vi "HFRR ADV v015 new software.vi"() -> ()   [LabVIEW 2025] (continued)
            n3529 = property class="DigNum (strict)"("Numeric Text.Text Colors:BG Color"="NC BG") -> ()  [unwired: 2 in, 2 out]
            n3530 = property class="DigNum (strict)"("Numeric Text.Text Colors:BG Color"="NC BG") -> ()  [unwired: 2 in, 2 out]
            n3531 = property class="DigNum (strict)"("Numeric Text.Text Colors:BG Color"="NC BG") -> ()  [unwired: 2 in, 2 out]
            n3532 = property class="DigNum (strict)"("Numeric Text.Text Colors:BG Color"="NC BG") -> ()  [unwired: 2 in, 2 out]
            n3533 = property class="DigNum (strict)"("Numeric Text.Text Colors:BG Color"="NC BG") -> ()  [unwired: 2 in, 2 out]
            n3534 = property class="DigNum (strict)"("Numeric Text.Text Colors:BG Color"="NC BG") -> ()  [unwired: 2 in, 2 out]
            n3535 = property class="DigNum (strict)"("Numeric Text.Text Colors:BG Color"="NC BG") -> ()  [unwired: 2 in, 2 out]
            n3536 = property class="DigNum (strict)"("Numeric Text.Text Colors:BG Color"="NC BG") -> ()  [unwired: 2 in, 2 out]
            n3537 = property class="DigNum (strict)"("Numeric Text.Text Colors:BG Color"="NC BG") -> ()  [unwired: 2 in, 2 out]
            n3538 = property class="DigNum (strict)"("Numeric Text.Text Colors:BG Color"="NC BG") -> ()  [unwired: 2 in, 2 out]
            n3539 = property class="DigNum (strict)"("Numeric Text.Text Colors:BG Color"="NC BG") -> ()  [unwired: 2 in, 2 out]
            n3540 = property on="FILE" class="Str"("Text.Text Colors:BG Color"="SC BG 3") -> ()  [unwired: 2 in, 2 out]
            n3541 = property on="Fuel Discription :" class="Str"("Text.Text Colors:BG Color"="SC BG 3") -> ()  [unwired: 2 in, 2 out]
            n3542 = property on="tested by" class="Str"("Text.Text Colors:BG Color"="SC BG 3") -> ()  [unwired: 2 in, 2 out]
            n3543 = property on="Remarks :" class="Str"("Text.Text Colors:BG Color"="SC BG 3") -> ()  [unwired: 2 in, 2 out]
            n3544 = property class="DigNum (strict)"("Numeric Text.Text Colors:Text Color"="NC Text") -> ()  [unwired: 2 in, 2 out]
            n3545 = property class="DigNum (strict)"("Numeric Text.Text Colors:Text Color"="NC Text") -> ()  [unwired: 2 in, 2 out]
            n3546 = property class="DigNum (strict)"("Numeric Text.Text Colors:Text Color"="NC Text") -> ()  [unwired: 2 in, 2 out]
            n3547 = property class="DigNum (strict)"("Numeric Text.Text Colors:Text Color"="NC Text") -> ()  [unwired: 2 in, 2 out]
            n3548 = property class="DigNum (strict)"("Numeric Text.Text Colors:Text Color"="NC Text") -> ()  [unwired: 2 in, 2 out]
            n3549 = property class="DigNum (strict)"("Numeric Text.Text Colors:Text Color"="NC Text") -> ()  [unwired: 2 in, 2 out]
            n3550 = property class="DigNum (strict)"("Numeric Text.Text Colors:Text Color"="NC Text") -> ()  [unwired: 2 in, 2 out]
            n3551 = property class="DigNum (strict)"("Numeric Text.Text Colors:Text Color"="NC Text") -> ()  [unwired: 2 in, 2 out]
            n3552 = property class="DigNum (strict)"("Numeric Text.Text Colors:Text Color"="NC Text") -> ()  [unwired: 2 in, 2 out]
            n3553 = property class="DigNum (strict)"("Numeric Text.Text Colors:Text Color"="NC Text") -> ()  [unwired: 2 in, 2 out]
            n3554 = property class="DigNum (strict)"("Numeric Text.Text Colors:Text Color"="NC Text") -> ()  [unwired: 2 in, 2 out]
            n3555 = property class="DigNum (strict)"("Numeric Text.Text Colors:Text Color"="NC Text") -> ()  [unwired: 2 in, 2 out]
            n3556 = property class="DigNum (strict)"("Numeric Text.Text Colors:Text Color"="NI Text  2") -> ()  [unwired: 2 in, 2 out]
            n3557 = property class="DigNum (strict)"("Numeric Text.Text Colors:Text Color"="NI Text  2") -> ()  [unwired: 2 in, 2 out]
            n3558 = property class="DigNum (strict)"("Numeric Text.Text Colors:Text Color"="NI Text  2") -> ()  [unwired: 2 in, 2 out]
            n3559 = property class="DigNum (strict)"("Numeric Text.Text Colors:Text Color"="NI Text  2") -> ()  [unwired: 2 in, 2 out]
            n3560 = property class="DigNum (strict)"("Numeric Text.Text Colors:Text Color"="NI Text  2") -> ()  [unwired: 2 in, 2 out]
            n3561 = property class="DigNum (strict)"("Numeric Text.Text Colors:Text Color"="NI Text  2") -> ()  [unwired: 2 in, 2 out]
            n3562 = property class="DigNum (strict)"("Numeric Text.Text Colors:Text Color"="NI Text  2") -> ()  [unwired: 2 in, 2 out]
            n3563 = property class="DigNum (strict)"("Numeric Text.Text Colors:Text Color"="NI Text  2") -> ()  [unwired: 2 in, 2 out]
            n3564 = property class="DigNum (strict)"("Numeric Text.Text Colors:Text Color"="NI Text  2") -> ()  [unwired: 2 in, 2 out]
            n3565 = property class="DigNum (strict)"("Numeric Text.Text Colors:Text Color"="NI Text  2") -> ()  [unwired: 2 in, 2 out]
            n3566 = property class="DigNum (strict)"("Numeric Text.Text Colors:Text Color"="NI Text  2") -> ()  [unwired: 2 in, 2 out]
            n3567 = property class="DigNum (strict)"("Numeric Text.Text Colors:Text Color"="NI Text  2") -> ()  [unwired: 2 in, 2 out]
            n3568 = property class="DigNum (strict)"("Numeric Text.Text Colors:Text Color"="NI Text  2") -> ()  [unwired: 2 in, 2 out]
            n3569 = property class="DigNum (strict)"("Numeric Text.Text Colors:Text Color"="NI Text  2") -> ()  [unwired: 2 in, 2 out]
            n3570 = property class="DigNum (strict)"("Numeric Text.Text Colors:Text Color"="NI Text  2") -> ()  [unwired: 2 in, 2 out]
            n3571 = property on="Coefficient Of Friction" class="XYGraph (strict)"("Plot Area:Colors:FG Color"="GFG  2", "Plot Area:Colors:BG Color"="GBG   2") -> ()  [unwired: 2 in, 2 out]
            n3572 = property on="Humidity ( %RH )" class="XYGraph (strict)"("Plot Area:Colors:FG Color"="GFG  2", "Plot Area:Colors:BG Color"="GBG   2") -> ()  [unwired: 2 in, 2 out]
            n3573 = property on="Air Temperature  ( °C )" class="XYGraph (strict)"("Plot Area:Colors:FG Color"="GFG  2", "Plot Area:Colors:BG Color"="GBG   2") -> ()  [unwired: 2 in, 2 out]
            n3574 = property on="Sample Temperature ( °C )" class="XYGraph (strict)"("Plot Area:Colors:FG Color"="GFG  2", "Plot Area:Colors:BG Color"="GBG   2") -> ()  [unwired: 2 in, 2 out]
            n3575 = property class="DigNum (strict)"("Numeric Text.Text Colors:BG Color"="NI BG 2") -> ()  [unwired: 2 in, 2 out]
            n3576 = property class="DigNum (strict)"("Numeric Text.Text Colors:BG Color"="NI BG 2") -> ()  [unwired: 2 in, 2 out]
            n3577 = property class="DigNum (strict)"("Numeric Text.Text Colors:BG Color"="NI BG 2") -> ()  [unwired: 2 in, 2 out]
            n3578 = property class="DigNum (strict)"("Numeric Text.Text Colors:BG Color"="NI BG 2") -> ()  [unwired: 2 in, 2 out]
            n3579 = property class="DigNum (strict)"("Numeric Text.Text Colors:BG Color"="NI BG 2") -> ()  [unwired: 2 in, 2 out]
            n3580 = property class="DigNum (strict)"("Numeric Text.Text Colors:BG Color"="NI BG 2") -> ()  [unwired: 2 in, 2 out]
            n3581 = property class="DigNum (strict)"("Numeric Text.Text Colors:BG Color"="NI BG 2") -> ()  [unwired: 2 in, 2 out]
            n3582 = property class="DigNum (strict)"("Numeric Text.Text Colors:BG Color"="NI BG 2") -> ()  [unwired: 2 in, 2 out]
            n3583 = property class="DigNum (strict)"("Numeric Text.Text Colors:BG Color"="NI BG 2") -> ()  [unwired: 2 in, 2 out]
            n3584 = property class="DigNum (strict)"("Numeric Text.Text Colors:BG Color"="NI BG 2") -> ()  [unwired: 2 in, 2 out]
            n3585 = property class="DigNum (strict)"("Numeric Text.Text Colors:BG Color"="NI BG 2") -> ()  [unwired: 2 in, 2 out]
            n3586 = property class="DigNum (strict)"("Numeric Text.Text Colors:BG Color"="NI BG 2") -> ()  [unwired: 2 in, 2 out]
            n3587 = property class="DigNum (strict)"("Numeric Text.Text Colors:BG Color"="NI BG 2") -> ()  [unwired: 2 in, 2 out]
            n3588 = property class="DigNum (strict)"("Numeric Text.Text Colors:BG Color"="NI BG 2") -> ()  [unwired: 2 in, 2 out]
            n3589 = property class="DigNum (strict)"("Numeric Text.Text Colors:BG Color"="NI BG 2") -> ()  [unwired: 2 in, 2 out]
            n3590 = property class="Bool"("Colors [4]"="Boolean BC T & BG") -> ()  [unwired: 2 in, 2 out]
            n3591 = property on="Save & Continue" class="Bool (strict)"("Colors [4]"="Boolean BC T & BG") -> ()  [unwired: 2 in, 2 out]
            n3592 = property on="Heater Button" class="Bool (strict)"("Colors [4]"="Boolean BC T & BG") -> ()  [unwired: 2 in, 2 out]
            n3593 = property class="Bool"("Colors [4]"="Boolean BC T & BG") -> ()  [unwired: 2 in, 2 out]
            n3594 = property on="Humidity" class="Bool (strict)"("Colors [4]"="Boolean BC T & BG") -> ()  [unwired: 2 in, 2 out]
            n3595 = property class="Bool (strict)"("Colors [4]"="Boolean BC T & BG") -> ()  [unwired: 2 in, 2 out]
            n3596 = property on="RUN" class="Bool (strict)"("Colors [4]"="Boolean BC T & BG") -> ()  [unwired: 2 in, 2 out]
            n3597 = property on="trip1 8" class="Bool (strict)"("Colors [4]"="Boolean BC T & BG") -> ()  [unwired: 2 in, 2 out]
            n3598 = property class="Bool"("Colors [4]"="Boolean BC T & BG") -> ()  [unwired: 2 in, 2 out]
            n3599 = property class="Bool (strict)"("Colors [4]"="Boolean BC T & BG") -> ()  [unwired: 2 in, 2 out]
            n3600 = property on="OPEN 1" class="Bool (strict)"("Colors [4]"="Boolean BC T & BG 2") -> ()  [unwired: 2 in, 2 out]
            n3601 = property on="OPEN 2" class="Bool (strict)"("Colors [4]"="Boolean BC T & BG 2") -> ()  [unwired: 2 in, 2 out]
            n3602 = property on="OPEN 3" class="Bool (strict)"("Colors [4]"="Boolean BC T & BG 2") -> ()  [unwired: 2 in, 2 out]
            n3603 = property on="OPEN 4" class="Bool (strict)"("Colors [4]"="Boolean BC T & BG 2") -> ()  [unwired: 2 in, 2 out]
            n3604 = property on="OPEN" class="Bool (strict)"("Colors [4]"="Boolean BC T & BG 2") -> ()  [unwired: 2 in, 2 out]
            n3605 = property on="rstv2" class="Bool"("Colors [4]"="Boolean BC T & BG 2") -> ()  [unwired: 2 in, 2 out]
            n3606 = property on="RST CP" class="Bool"("Colors [4]"="Boolean BC T & BG 2") -> ()  [unwired: 2 in, 2 out]
            n3607 = property on="RSTV1 3" class="Bool"("Colors [4]"="Boolean BC T & BG 2") -> ()  [unwired: 2 in, 2 out]
            n3608 = property on="RSTV1 2" class="Bool"("Colors [4]"="Boolean BC T & BG 2") -> ()  [unwired: 2 in, 2 out]
          }
          frame #1 {
          }
        }
        n3609 = local read "Quit"() -> (w4479:bool)
      }
    }
    frame Enabled {
    }
  }
  n3610 = while {
    shift-right: [w4497] -> _
    shift-left: _ -> [w4498]
    shift-right: [w4495] -> _
    shift-left: T19 {"Read Heave and Surge"="", "Bytes at Heave Port"=0.0, "Heave and Surge COM Port:"="COM9", "Com Port 2"="COM7", "Residual Due"="", "Heave COM Status 2"=TRUE, "Heave COM Status"=TRUE, "Port 2"=TRUE, "Sway PPR"=6400.0, "Surge PPR"=6400.0, "Heave PPR"=6400.0, "Sway Pitch"=2.0, "Surge Pitch"=3.0, "Heave Pitch"=4.0, "Sway Pulses/mm"=320.0, "Surge Pulses/mm"=1600.0, "Heave Pulses/mm"=1600.0, "inner loop"=0.0, "Read Heave and Surge 2"="", "String 36"="", "Write S"=FALSE, "WriteCC1"=[""], "Heave COM Loop"=0, "LastCom"="", "EXIT"=FALSE, "Error Heave"={"status"=TRUE, "code"=-1073807343, "source"=""}} -> [w4494]
    shift-right: [w4492] -> _
    shift-left: enum16{"init", "MAIN", "Panel Close"}."init" -> [w4493]
    stop <- w4496 stop-if-true
    n3611 = case shown="\"MAIN\"" w4493 {
      tunnel: w4498 -> [w4512 w4527 w4588 w4590]
      tunnel: [w4506 w4536 w4588 w4590] -> w4497
      tunnel: [_ _ TRUE _] -> w4496
      tunnel: [w4502 w4533 w4586 w4589] -> w4495
      tunnel: w4494 -> [w4509 w4526 w4586 w4589]
      tunnel: [enum16{"init", "MAIN", "Panel Close"}."MAIN" w4520 _ _] -> w4492
      frame "init" {
        n3612 = Bundle By Name(cluster=w4509, "Heave and Surge COM Port:"="C3 :") -> (w4508:T19)
        n3613 = call "Instrument fgv.vi"("Enum"=T31."INIT", "error in (no error) 2"=w4512, "INPUT"=w4508) -> ("error"=w4510:errorcluster, "output"=w4505:T19)  [unwired: 6 in, 1 out]
        n3614 = case shown="Error" w4510 {
          selector: w4510 -> [w4514 _]
          tunnel: [w4514 w4518] -> w4506
          tunnel: w4505 -> [w4513 w4516]
          tunnel: [w4513 w4515] -> w4503
          frame No Error {
          }
          frame Error {
            n3615 = call "Instrument fgv.vi"("Enum"=T31."ERROR INIT", "INPUT"=w4516) -> ("error"=w4519:errorcluster, "output"=w4515:T19)  [unwired: 7 in, 1 out]
            n3616 = call <vilib>:"Clear Errors.vi"("error in (no error)"=w4519) -> ("error out"=w4518:errorcluster)  [unwired: 5 in, 1 out]
          }
        }
        n3617 = local read "LastCom"() -> (w4501:string)
        n3618 = Unbundle By Name(w4503) -> ("Heave COM Status 2"=→"COM Status" →"Instrument Status":bool, "Error Heave"=→"Error":errorcluster)  [unwired: 1 out]
        n3619 = Bundle By Name(cluster=w4503, "LastCom"=w4501) -> (w4502:T19)
      }
      frame "MAIN" {
        n3620 = Unbundle By Name(w4526) -> ("Com Port 2"=w4538:refnum<visa-resource-name>)
        n3621 = local write "Com Port 4"(w4538) -> ()
        n3622 = local read "C3 :"() -> (w4524:refnum<visa-resource-name>)
        n3623 = Bundle By Name(cluster=w4526, "Heave and Surge COM Port:"=w4524) -> (w4525:T19)
        n3624 = Equal?(x=w4538, y=w4524) -> (x = y?=w4537:bool)
        n3625 = case shown="True" w4537 {
          tunnel: [w4542 w4559] -> w4536
          tunnel: w4527 -> [w4543 w4565]
          tunnel: w4525 -> [w4541 w4563]
          tunnel: [w4540 w4558] -> w4533
          frame False {
            n3626 = call <vilib>:"Clear Errors.vi"("error in (no error)"=w4543) -> ("error out"=w4539:errorcluster)  [unwired: 5 in, 1 out]
            n3627 = call "Instrument fgv.vi"("Enum"=T31."ERROR INIT", "error in (no error) 2"=w4539, "INPUT"=w4541) -> ("error"=w4545:errorcluster, "output"=w4540:T19)  [unwired: 6 in, 1 out]
            n3628 = call <vilib>:"Clear Errors.vi"("error in (no error)"=w4545) -> ("error out"=w4542:errorcluster)  [unwired: 5 in, 1 out]
          }
          frame True {
            n3629 = call "Instrument fgv.vi"("Enum"=T31."READ", "error in (no error) 2"=w4565, "INPUT"=w4563) -> ("error"=w4564:errorcluster, "output"=w4555:T19)  [unwired: 6 in, 1 out]
            n3630 = Bundle By Name(cluster=w4555, "String 36"="String 11") -> (w4554:T19)
            n3631 = case shown="True" "Write S" {
              selector: "Write S" -> [_ w4585]
              tunnel: w4564 -> [w4578 w4584]
              tunnel: [w4578 w4583] -> w4551
              tunnel: w4554 -> [w4577 w4580]
              tunnel: [w4577 w4579] -> w4550
              frame False {
              }
              frame True {
                n3632 = Not(x=w4585) -> (.not. x?=w4581:bool)
                n3633 = local write "Write S"(w4581) -> ()
                n3634 = call "Instrument fgv.vi"("Enum"=T31."MANUAL WRITE", "error in (no error) 2"=w4584, "INPUT"=w4580) -> ("error"=w4583:errorcluster, "output"=w4579:T19)  [unwired: 6 in, 1 out]
              }
            }
            n3635 = Array Size(array="WriteHumidity") -> (size(s)=w4548:i32)
            n3636 = Greater Than 0?(x=w4548) -> (x > 0?=w4546:bool)
            n3637 = call "Instrument fgv.vi"("Enum"=T31."WRITE", "error in (no error) 2"=w4551, "WriteCC1"="WriteHumidity", "INPUT"=w4550) -> ("error"=w4561:errorcluster, "WriteCC1 2"=w4549:string[], "output"=w4560:T19)  [unwired: 5 in]
            n3638 = case shown="True" w4546 {
              tunnel: w4549 -> [_ w4567]
              frame False {
              }
              frame True {
                n3639 = local write "WriteHumidity"(w4567) -> ()
              }
            }
            n3640 = case shown="Error" w4561 {
              selector: w4561 -> [w4568 w4571]
              tunnel: w4560 -> [w4569 w4576]
              tunnel: [w4569 w4575] -> w4558
              tunnel: [w4568 w4573] -> w4559
              frame No Error {
              }
              frame Error {
                n3641 = call <vilib>:"Clear Errors.vi"("error in (no error)"=w4571) -> ("error out"=w4570:errorcluster)  [unwired: 5 in, 1 out]
                n3642 = call "Instrument fgv.vi"("Enum"=T31."ERROR INIT", "error in (no error) 2"=w4570, "INPUT"=w4576) -> ("error"=w4574:errorcluster, "output"=w4575:T19)  [unwired: 6 in, 1 out]
                n3643 = call <vilib>:"Clear Errors.vi"("error in (no error)"=w4574) -> ("error out"=w4573:errorcluster)  [unwired: 5 in, 1 out]
              }
            }
            n3644 = Unbundle By Name(w4558) -> ("LastCom"=→"LastCom":string, "Read Heave and Surge"=→"Read Humidity":string)
          }
        }
        n3645 = Unbundle By Name(w4533) -> ("Heave COM Status 2"=w4535:bool, "Heave COM Status"=w4534:bool, "Error Heave"=w4531:errorcluster, "Bytes at Heave Port"=→"Bytes at Humidity Port":dbl)
        n3646 = Unbundle By Name(w4531) -> ("status"=→"Humidity Port":bool)
        n3647 = Not(x=w4534) -> (.not. x?=w4528:bool)
        n3648 = local write "Error"(w4531) -> ()
        n3649 = Not(x=w4535) -> (.not. x?=w4529:bool)
        n3650 = local write "Instrument Status"(w4528) -> ()
        n3651 = local write "COM Status"(w4529) -> ()
        n3652 = local read "Quit"() -> (w4521:bool)
        n3653 = Select(t=enum16{"init", "MAIN", "Panel Close"}."Panel Close", s=w4521, f=enum16{"init", "MAIN", "Panel Close"}."MAIN") -> (s? t:f=w4520:enum16{"init", "MAIN", "Panel Close"})
      }
      frame "Panel Close" {
      }
      frame Default {
      }
    }
  }
  n3654 = while {
    stop <- w4616 stop-if-true
    n3655 = local read "Read Humidity"() -> (w4597:string)
    n3656 = call <vilib>:"High Resolution Polling Wait.vi"("seconds to wait"=0.1) -> ()  [unwired: 10 in, 1 out]
    n3657 = Spreadsheet String To Array(delimiter (Tab)=",", format string="", spreadsheet string=w4597, array type (2D Dbl)=string[] []) -> (array=w4611:string[])
    n3658 = for {
      tunnel: w4611 -> [w4621] mode=indexing
      tunnel: string[] ["STATE;", "SET;", "RH;", "T;", "AMB_RH;", "AMB_T;", "PUMP;", "FAN_IN;", "FAN_OUT;", "DEHUM;", "CURRENT;", "STALL;"] -> [w4620] mode=indexing
      tunnel: [w4619] -> w4610 mode=indexing
      n3659 = Match Pattern(string=w4621, regular expression=w4620) -> (after substring=w4619:string)  [unwired: 1 in, 3 out]
    }
    n3660 = Index Array(array=w4610) -> (element #1=→"STATE :":string, element #2=→"SET :":string, element #3=w4599:string, element #4=→"T :":string, element #5=w4596:string, element #6=→"AMB_T :":string, element #7=→"PUMP :":string, element #8=→"FAN_IN :":string, element #9=→"FAN_OUT :":string, element #10=→"DEHUM :":string, element #11=→"CURRENT :":string, element #12=→"STALL :":string)  [unwired: 12 in]
    "RH :" <- w4599
    "AMB_RH :" <- w4596
    n3661 = Fract/Exp String To Number(string=w4599) -> (number=w4591:dbl)  [unwired: 3 in, 1 out]
    n3662 = Fract/Exp String To Number(string=w4596) -> (number=w4595:dbl)  [unwired: 3 in, 1 out]
    n3663 = local write "Ambient Humidity :"(w4595) -> ()
    n3664 = Equal?(x=w4591, y=0.0) -> (x = y?=w4593:bool)
    n3665 = case shown="True" w4593 {
      tunnel: [w4617 w4618] -> w4592
      tunnel: w4591 -> [w4617 _]
      frame False {
        (unwired) 0.0
        "Humidity temp" <- w4617
      }
      frame True {
        n3666 = local read "Humidity temp"() -> (w4618:dbl)
      }
    }
    "RH Numeric:" <- w4592
    n3667 = local read "Quit"() -> (w4616:bool)
  }
  n3668 = disable-structure shown="Disabled" {
    frame Disabled {
      n3669 = while {
        tunnel: [w4855] -> _
        i -> [w4855]
        stop <- w4852 stop-if-true
        n3670 = local read "powstat"() -> (w4853:bool)
        n3671 = case shown="True" w4853 {
          frame False {
          }
          frame True {
            n3672 = local read "RUN"() -> (w4856:bool)
            n3673 = case shown="True" w4856 {
              frame False {
                w4886 = 65.0 ("y")
                n3674 = local read "Set Hz"() -> (w4914:dbl)
                n3675 = local read "NORMAL LOAD"() -> (w4915:dbl)
                n3676 = Multiply(x=w4914, y=60.0) -> (x*y=w4921:dbl)
                n3677 = Multiply(x=1.2 ("y"), y=0.949) -> (x*y=w4890:dbl)
                n3678 = Multiply(x=1.2 ("y"), y=0.8166) -> (x*y=w4894:dbl)
                n3679 = Multiply(x=1.2 ("y"), y=0.851) -> (x*y=w4889:dbl)
                n3680 = local read "FF 2"() -> (w4913:dbl)
                n3681 = Absolute Value(x=w4921) -> (abs(x)=w4919:dbl)
                n3682 = case shown="13.." w4913 {
                  tunnel: [1 2 3] -> w4911
                  frame 0..10, Default {
                    # "Normal"
                  }
                  frame 11, 12 {
                  }
                  frame 13.. {
                  }
                }
                "FF STATE" <- w4911
                n3683 = local read "TEMP"() -> (w4874:dbl)
                n3684 = local read item#-1() -> (w4888)
                n3685 = Less?(x=w4888, y=w4894) -> (x < y?=w4891:bool)
                n3686 = In Range and Coerce(upper limit=w4890, x=w4888, lower limit=w4889) -> (In Range?=w4892:bool)  [unwired: 1 out]
                n3687 = case shown="3601.." w4919 {
                  tunnel: [1 2 3] -> w4917
                  frame 0..3000, Default {
                    # "Normal"
                  }
                  frame 3001..3600 {
                  }
                  frame 3601.. {
                  }
                }
                n3688 = case shown="11.." w4915 {
                  tunnel: [1 3] -> w4916
                  frame 1..10, Default {
                  }
                  frame 11.. {
                  }
                }
                "NL STATE" <- w4916
                n3689 = Multiply(x=1.2 ("y"), y=0.95) -> (x*y=w4904:dbl)
                n3690 = Multiply(x=w4886, y=0.954) -> (x*y=w4878:dbl)
                n3691 = Or(x=w4891, y=w4892) -> (x .or. y?=w4893:bool)
                n3692 = Greater Or Equal?(x=w4888, y=w4904) -> (x >= y?=w4901:bool)
                n3693 = Multiply(x=w4886, y=0.99) -> (x*y=w4875:dbl)
                n3694 = Greater Or Equal?(x=w4874, y=w4875) -> (x >= y?=w4880:bool)
                n3695 = Greater Or Equal?(x=w4874, y=w4878) -> (x >= y?=w4877:bool)
                n3696 = case shown="0, 1, Default" w4888 {
                  tunnel: [1 3] -> w4905
                  frame 0, 1, Default {
                  }
                  frame 2.. {
                  }
                }
                n3697 = case shown="True" w4901 {
                  tunnel: [1 3] -> w4906
                  frame False {
                  }
                  frame True {
                  }
                }
                n3698 = case shown="True" w4893 {
                  tunnel: [1 2] -> w4907
                  frame False {
                  }
                  frame True {
                  }
                }
                n3699 = case shown="..0" w4874 {
                  tunnel: [2 3 3 1] -> w4881
                  frame 61, 62 {
                  }
                  frame 63.. {
                  }
                  frame ..0 {
                  }
                  frame 10..60, Default {
                  }
                }
                n3700 = case shown="True" w4880 {
                  tunnel: [1 3] -> w4882
                  frame False {
                  }
                  frame True {
                  }
                }
                n3701 = Number To Decimal String(number=w4917) -> (decimal integer string=w4918:string)  [unwired: 1 in]
                n3702 = case shown="True" w4877 {
                  tunnel: [1 2] -> w4883
                  frame False {
                  }
                  frame True {
                  }
                }
                n3703 = Number To Decimal String(number=1) -> (decimal integer string=→"Air temp":string)  [unwired: 1 in]
                n3704 = Number To Decimal String(number=w4911) -> (decimal integer string=→"ff_st":string)  [unwired: 1 in]
                n3705 = local write "sp_st"(w4918) -> ()
                n3706 = Number To Decimal String(number=w4916) -> (decimal integer string=→"nl_st":string)  [unwired: 1 in]
                n3707 = Build Array(w4881, w4882, w4883) -> (w4884:i32[])
                n3708 = Build Array(w4905, w4906, w4907) -> (w4908:i32[])
                n3709 = Array Max & Min(array=w4884) -> (max value=w4885:i32)  [unwired: 3 out]
                n3710 = Array Max & Min(array=w4908) -> (max value=w4909:i32)  [unwired: 3 out]
                n3711 = Number To Decimal String(number=w4885) -> (decimal integer string=w4873:string)  [unwired: 1 in]
                n3712 = Number To Decimal String(number=w4909) -> (decimal integer string=→"Stroke Ln 2":string)  [unwired: 1 in]
                n3713 = local write "temp_st"(w4873) -> ()
              }
              frame True {
                w4971 = 65.0 ("y")
                # "Healthy -1\nWarning -2\nError -3"
                n3714 = local read "TEMP"() -> (w4982:dbl)
                n3715 = local read "NORMAL LOAD"() -> (w4986:dbl)
                n3716 = local read "Set Hz"() -> (w4984:dbl)
                n3717 = Multiply(x=1.2 ("y"), y=0.949) -> (x*y=w4966:dbl)
                n3718 = Multiply(x=1.2 ("y"), y=0.8166) -> (x*y=w4962:dbl)
                n3719 = Multiply(x=1.2 ("y"), y=0.851) -> (x*y=w4967:dbl)
                n3720 = Multiply(x=w4971, y=0.954) -> (x*y=w4978:dbl)
                n3721 = Multiply(x=w4971, y=0.99) -> (x*y=w4981:dbl)
                n3722 = Greater Or Equal?(x=w4982, y=w4981) -> (x >= y?=w4976:bool)
                n3723 = Multiply(x=w4984, y=60.0) -> (x*y=w4990:dbl)
                n3724 = Greater Or Equal?(x=w4982, y=w4978) -> (x >= y?=w4979:bool)
                n3725 = local read "FF 2"() -> (w4985:dbl)
                n3726 = local read item#-1() -> (w4968)
                n3727 = Less?(x=w4968, y=w4962) -> (x < y?=w4965:bool)
                n3728 = In Range and Coerce(upper limit=w4966, x=w4968, lower limit=w4967) -> (In Range?=w4964:bool)  [unwired: 1 out]
                n3729 = Absolute Value(x=w4990) -> (abs(x)=w4988:dbl)
                n3730 = case shown="63.." w4982 {
                  tunnel: [2 3 3 1] -> w4975
                  frame 61, 62 {
                  }
                  frame 63.. {
                  }
                  frame ..0 {
                  }
                  frame 10..60, Default {
                  }
                }
                n3731 = case shown="True" w4976 {
                  tunnel: [1 3] -> w4974
                  frame False {
                  }
                  frame True {
                  }
                }
                n3732 = case shown="True" w4979 {
                  tunnel: [1 2] -> w4973
                  frame False {
                  }
                  frame True {
                  }
                }
                n3733 = Multiply(x=1.2 ("y"), y=0.95) -> (x*y=w4952:dbl)
                n3734 = case shown="1..10, Default" w4986 {
                  tunnel: [1 3] -> w4993
                  frame 1..10, Default {
                  }
                  frame 11.. {
                  }
                }
                n3735 = case shown="0..10, Default" w4985 {
                  tunnel: [1 2 3] -> w4992
                  frame 0..10, Default {
                  }
                  frame 11, 12 {
                  }
                  frame 13.. {
                  }
                }
                n3736 = case shown="3601.." w4988 {
                  tunnel: [1 2 3] -> w4987
                  frame 0..3000, Default {
                    # "Normal"
                  }
                  frame 3001..3600 {
                  }
                  frame 3601.. {
                  }
                }
                n3737 = Or(x=w4965, y=w4964) -> (x .or. y?=w4963:bool)
                n3738 = Greater Or Equal?(x=w4968, y=w4952) -> (x >= y?=w4955:bool)
                n3739 = case shown="0, 1, Default" w4968 {
                  tunnel: [1 3] -> w4951
                  frame 0, 1, Default {
                  }
                  frame 2.. {
                  }
                }
                n3740 = case shown="True" w4955 {
                  tunnel: [1 3] -> w4950
                  frame False {
                  }
                  frame True {
                  }
                }
                n3741 = case shown="True" w4963 {
                  tunnel: [1 2] -> w4949
                  frame False {
                  }
                  frame True {
                  }
                }
                n3742 = Build Array(w4975, w4974, w4973) -> (w4972:i32[])
                n3743 = Number To Decimal String(number=w4987) -> (decimal integer string=→"sp_st":string)  [unwired: 1 in]
                n3744 = Array Max & Min(array=w4972) -> (max value=w4969:i32)  [unwired: 3 out]
                "TEMP STATE" <- w4969
                n3745 = Number To Decimal String(number=w4993) -> (decimal integer string=w4996:string)  [unwired: 1 in]
                n3746 = Number To Decimal String(number=w4992) -> (decimal integer string=w4994:string)  [unwired: 1 in]
                n3747 = Number To Decimal String(number=w4969) -> (decimal integer string=→"temp_st":string)  [unwired: 1 in]
                n3748 = Build Array(w4951, w4950, w4949) -> (w4948:i32[])
                n3749 = local write "nl_st"(w4996) -> ()
                n3750 = local write "ff_st"(w4994) -> ()
                n3751 = Number To Decimal String(number=1) -> (decimal integer string=w4991:string)  [unwired: 1 in]
                n3752 = Array Max & Min(array=w4948) -> (max value=w4947:i32)  [unwired: 3 out]
                n3753 = local write "Air temp"(w4991) -> ()
                n3754 = Number To Decimal String(number=w4947) -> (decimal integer string=w4946:string)  [unwired: 1 in]
                n3755 = local write "Stroke Ln 2"(w4946) -> ()
              }
            }
            n3756 = local read "Stroke Ln 2"() -> (w4858:string)
            n3757 = local read "nl_st"() -> (w4864:string)
            n3758 = local read "ff_st"() -> (w4861:string)
            n3759 = local read "sp_st"() -> (w4862:string)
            n3760 = local read "temp_st"() -> (w4863:string)
            n3761 = local read "Air temp"() -> (w4857:string)
            n3762 = Replace Array Subset(array="in", new element #1=w4864, index #1=1 ("index"), new element #2=w4861, index #2=2 ("index"), new element #3=w4863, index #3=3 ("index"), new element #4=w4862, index #4=4 ("index"), new element #5=w4858, index #5=5 ("index"), new element #6=w4857, index #6=6 ("index"), new element #7="Sensor State" ("new element/subarray"), index #7=0 ("index")) -> (→"out":string[])
          }
        }
        n3763 = Wait (ms)(milliseconds to wait=u32 10) -> ()  [unwired: 1 out]
        n3764 = local read "Quit"() -> (w4852:bool)
      }
      n3765 = while {
        stop <- w4827 stop-if-true
        n3766 = local read "run replace"() -> (w4829:bool)
        n3767 = Wait (ms)(milliseconds to wait=u32 100) -> ()  [unwired: 1 out]
        n3768 = Equal?(x="FLAG 2", y=0.0) -> (x = y?=w4830:bool)
        n3769 = case shown="True" w4830 {
          frame False {
          }
          frame True {
            n3770 = local write "FLAG 2"(100.0 ("FLAG 2")) -> ()
            n3771 = call <vilib>:"Read Characters From File.vi"("file path (dialog if empty)"=path "C:/LAB-IQ-NXT/WO 2449 TT.sig", "convert eol? (no:F)"=FALSE ("append to file? (new file:F)")) -> ("character string"=w4833:string)  [unwired: 4 in, 3 out]
            n3772 = call <vilib>:"Read Characters From File.vi"("file path (dialog if empty)"=path "C:/LAB-IQ-NXT/WO 2449 TRH.sig", "convert eol? (no:F)"=FALSE ("append to file? (new file:F)")) -> ("character string"=w4834:string)  [unwired: 4 in, 3 out]
            n3773 = Decimal String To Number(string=w4833) -> (number=w4835:i32)  [unwired: 2 in, 1 out]
            n3774 = local write "Total No. of Tests"(w4835) -> ()
            n3775 = Decimal String To Number(string=w4834) -> (number=w4838:i32)  [unwired: 2 in, 1 out]
            n3776 = local write "SEN.RUN HRS"(w4838) -> ()
          }
        }
        n3777 = case shown="True" w4829 {
          frame False {
          }
          frame True {
            n3778 = Equal?(x="FLAG 4", y=0.0) -> (x = y?=w4842:bool)
            n3779 = case shown="False" w4842 {
              frame False {
                n3780 = Get Date/Time In Seconds() -> (seconds since 1Jan1904=w4848:timestamp)
                n3781 = local read "START 3"() -> (w4846:dbl)
                n3782 = To Double Precision Float(number=w4848) -> (double precision float=w4847:dbl)
                n3783 = Subtract(x=w4847, y=w4846) -> (x-y=→"SENSOR TIME":dbl)
              }
              frame True {
                n3784 = Get Date/Time In Seconds() -> (seconds since 1Jan1904=w4850:timestamp)
                n3785 = local write "FLAG 4"(100.0 ("FLAG")) -> ()
                n3786 = To Double Precision Float(number=w4850) -> (double precision float=→"START 3":dbl)
              }
            }
          }
        }
        n3787 = local read "Quit"() -> (w4827:bool)
      }
      n3788 = while {
        shift-right: [w4627] -> _
        shift-left: _ -> [w4628]
        tunnel: [w4623] -> _
        i -> [w4623]
        stop <- w4622 stop-if-true
        n3789 = Wait (ms)(milliseconds to wait=u32 50 ("Refresh Rate (ms)")) -> ()  [unwired: 1 out]
        n3790 = local read "Json End Flg"() -> (w4624:bool)
        n3791 = Not(x="Upld AR 2") -> ()  [unwired: 1 out]
        n3792 = local read "Upld AR 2"() -> (w4625:bool)
        n3793 = call "Elapsed Time9"("Time Target (s)"="Sen.Upload Rate (s)", "Reset"=FALSE, "Auto Reset"=TRUE) -> ("Time has Elapsed"=w4634:bool)  [unwired: 9 in, 7 out]
        n3794 = Or(x=w4634, y=w4624) -> (x .or. y?=w4630:bool)
        n3795 = case shown="True" w4630 {
          frame False {
          }
          frame True {
            w4726 = "\"SensorName\":\"" ("string")
            w4696 = " \"},{"
            w4721 = "\",\"SensorState\":\""
            w4723 = "\",\"SensorModelNumber\":\"" ("string")
            w4722 = "\",\"SensorRuntimeHours\":\"" ("string")
            n3796 = local read "model num"() -> (w4720:string[])
            n3797 = local read "Sensor name"() -> (w4739:string[])
            n3798 = local read "run"() -> (w4710:string[])
            n3799 = local read "SENSOR TIME"() -> (w4666:dbl)
            n3800 = local read "out"() -> (w4659:string[])
            n3801 = local read "Total No. of Tests"() -> (w4664:dbl)
            n3802 = Select(t=60.0, s="Run test 3", f=3600.0) -> (s? t:f=w4674:dbl)
            n3803 = Index Array(array=w4720, index #1=1 ("index")) -> (element #1=w4719:string, element #2=w4718:string, element #3=w4717:string, element #4=w4716:string, element #5=w4715:string, element #6=w4714:string)  [unwired: 5 in]
            n3804 = Index Array(array=w4710, index #1=1 ("index")) -> (element #1=w4709:string, element #2=w4708:string, element #3=w4707:string, element #4=w4706:string, element #5=w4705:string, element #6=w4704:string)  [unwired: 5 in]
            n3805 = Index Array(array=w4739, index #1=1 ("index")) -> (element #1=w4738:string, element #2=w4737:string, element #3=w4736:string, element #4=w4735:string, element #5=w4725:string, element #6=w4724:string)  [unwired: 5 in]
            n3806 = Index Array(array=w4659, index #1=1 ("index")) -> (element #1=w4691:string, element #2=w4690:string, element #3=w4689:string, element #4=w4688:string, element #5=w4687:string, element #6=w4686:string)  [unwired: 5 in]
            n3807 = local read "SEN.RUN HRS"() -> (w4662:dbl)
            n3808 = Divide(x=w4666, y=w4674) -> (x/y=w4673:dbl)
            n3809 = Increment(x=w4673) -> (x+1=w4669:dbl)
            n3810 = Number To Decimal String(number=w4669) -> (decimal integer string=→"run hrs":string)  [unwired: 1 in]
            n3811 = Divide(x=w4662, y=3600.0 ("f")) -> (x/y=w4657:dbl)
            n3812 = Round To Nearest(number=w4657) -> (nearest integer value=w4655:dbl)
            n3813 = Number To Decimal String(number=w4655) -> (decimal integer string=w4656:string)  [unwired: 1 in]
            n3814 = Number To Decimal String(number=w4664) -> (decimal integer string=w4665:string)  [unwired: 1 in]
            n3815 = local read "Model No"() -> (w4670:string)
            n3816 = local read "UUID"() -> (w4765:string)
            n3817 = local read "Serial No"() -> (w4769:string)
            n3818 = local read "Secret Key"() -> (w4770:string)
            n3819 = Concatenate Strings("\",\"MachineSerialNumber\":\"" ("string"), w4769) -> (w4773:string)
            n3820 = Concatenate Strings("\",\"ModelNumber\":\"" ("string"), w4670) -> (w4671:string)
            n3821 = Concatenate Strings("\",\"MachineRuntimeHours\":\"" ("string"), w4656) -> (w4774:string)
            n3822 = Concatenate Strings("\",\"MachineRuntimeCycles\":\"", w4665) -> (w4767:string)
            n3823 = Concatenate Strings(w4723, w4719) -> (w4753:string)
            n3824 = Concatenate Strings(w4722, w4709) -> (w4754:string)
            n3825 = Concatenate Strings(w4721, w4691) -> (w4752:string)
            n3826 = Concatenate Strings(w4773, w4671, w4774, w4767) -> (w4776:string)
            n3827 = Concatenate Strings(w4723, w4718) -> (w4750:string)
            n3828 = Concatenate Strings(w4722, w4708) -> (w4749:string)
            n3829 = Concatenate Strings(w4721, w4690) -> (w4751:string)
            n3830 = Concatenate Strings(w4723, w4717) -> (w4745:string)
            n3831 = Concatenate Strings(w4722, w4707) -> (w4746:string)
            n3832 = Concatenate Strings(w4721, w4689) -> (w4744:string)
            n3833 = Concatenate Strings(w4723, w4716) -> (w4742:string)
            n3834 = Concatenate Strings(w4722, w4706) -> (w4741:string)
            n3835 = Concatenate Strings(w4721, w4688) -> (w4743:string)
            n3836 = Concatenate Strings(w4753, w4754, w4752) -> (w4755:string)
            n3837 = Concatenate Strings(w4723, w4715) -> (w4732:string)
            n3838 = Concatenate Strings(w4722, w4705) -> (w4733:string)
            n3839 = Concatenate Strings(w4723, w4714) -> (w4729:string)
            n3840 = Concatenate Strings(w4722, w4704) -> (w4728:string)
            n3841 = Concatenate Strings(w4721, w4687) -> (w4731:string)
            n3842 = Concatenate Strings(w4721, w4686) -> (w4730:string)
            n3843 = Concatenate Strings("{\"SecretKey\":\"", w4770, w4776, "\",\"UUID\" : \"", w4765, "\",\"SensorInformation\":", "[{" ("string")) -> (w4703:string)
            n3844 = Concatenate Strings(w4750, w4749, w4751) -> (w4748:string)
            n3845 = Concatenate Strings(w4745, w4746, w4744) -> (w4747:string)
            n3846 = Concatenate Strings(w4742, w4741, w4743) -> (w4740:string)
            n3847 = Concatenate Strings(w4732, w4733, w4731) -> (w4734:string)
            n3848 = Concatenate Strings(w4729, w4728, w4730) -> (w4727:string)
            n3849 = Concatenate Strings(w4726, w4738, w4755, w4696) -> (w4702:string)
            n3850 = Concatenate Strings(w4726, w4737, w4748, w4696) -> (w4701:string)
            n3851 = Concatenate Strings(w4726, w4736, w4747, w4696) -> (w4700:string)
            n3852 = Concatenate Strings(w4726, w4735, w4740, w4696) -> (w4699:string)
            n3853 = Concatenate Strings(w4726, w4725, w4734, w4696) -> (w4698:string)
            n3854 = Concatenate Strings(w4726, w4724, w4727, "\"}" ("string")) -> (w4697:string)
            n3855 = Concatenate Strings(w4703, w4702, w4701, w4700, w4699, w4698, w4697, "]}" ("string")) -> (w4694:string)
            n3856 = local read "SEN.RUN HRS"() -> (w4661:dbl)
            n3857 = disable-structure shown="Disabled" {
              frame Disabled {
                n3858 = local read "state"() -> (w4780:string[])
                n3859 = Delete From Array(array=w4780, index=0) -> (array with subset deleted=w4778:string[])  [unwired: 1 in, 1 out]
                n3860 = for {
                  N: 6 -> [_]
                  tunnel: w4778 -> [w4791] mode=indexing
                  tunnel: [w4790] -> w4777 mode=indexing
                  n3861 = Equal?(x=w4791, y="Warning") -> (x = y?=w4787:bool)
                  n3862 = Equal?(x=w4791, y="Healthy") -> (x = y?=w4784:bool)
                  n3863 = Select(t="2" ("y"), s=w4787, f="3" ("y")) -> (s? t:f=w4782:string)
                  n3864 = Select(t="1" ("y"), s=w4784, f=w4782) -> (s? t:f=w4790:string)
                }
                "state1" <- w4777
              }
              frame Enabled {
              }
            }
            n3865 = stacked-sequence {
              tunnel: w4694 -> [w4802 _ _]
              tunnel: [_ _ w4818] -> _
              frame #0 {
                (unwired) FALSE ("convert eol (F)")
                w4804 = enum16{"start", "end", "current"}."start" ("pos mode (0:2)")
                n3866 = local read "Path"() -> (w4798:path)
                n3867 = Path To String(path=w4798) -> (string=w4810:string)
                n3868 = Concatenate Strings(w4810, "\\", "Sensor File Name") -> (w4811:string)
                n3869 = local write "standard output 2"(" ") -> ()
                n3870 = String To Path(string=w4811) -> (path=w4801:path)
                n3871 = call <vilib>:"Open_Create_Replace File.vi"("advisory dialog? (display:T)"=FALSE, "function (open:0)"=T32."create or replace", "file path"=w4801) -> ("error out"=w4814:errorcluster, "refnum"=w4813:refnum<file>)  [unwired: 5 in, 2 out]
                n3872 = Set File Position(refnum=w4813, from (0:start)=w4804, error in=w4814) -> (refnum out=w4794:refnum<file>, error out=w4793:errorcluster)  [unwired: 1 in]
                n3873 = Write to Binary File(file (use dialog)=w4794, data=" ", error in=w4793, 5:FALSE ("prepend array or string size? (T)")) -> (refnum out=w4805:refnum<file>, error out=w4806:errorcluster)  [unwired: 2 in, 1 out]
                n3874 = Set File Position(offset (in bytes) (0)=w4804, refnum=w4805, error in=w4806) -> (refnum out=w4797:refnum<file>, error out=w4796:errorcluster)  [unwired: 1 in]
                n3875 = Write to Binary File(file (use dialog)=w4797, data=w4802, error in=w4796, 5:FALSE ("prepend array or string size? (T)")) -> (error out=w4800:errorcluster)  [unwired: 2 in, 2 out]
                n3876 = flat-sequence {
                  tunnel: w4801 -> [w4816]
                  tunnel: w4800 -> [_]
                  frame #0 {
                    n3877 = call <vilib>:"Read Characters From File.vi"("file path (dialog if empty)"=w4816) -> ("character string"=→"Sensor Health JSON string":string)  [unwired: 5 in, 3 out]
                  }
                }
                "SinglePoint  2" <- w4802
              }
              frame #1 {
              }
              frame #2 {
                (unwired) "\"Stored\": true" ("string")
                n3878 = call <vilib>:"System Exec.vi"("run minimized? (F)"=TRUE, "wait until completion? (T)"=TRUE, "working directory"=path "C:/LAB-IQ-NXT", "command line"="C:\\LAB-IQ-NXT\\JPostH.bat") -> ("standard error"=→"Respose From Server 2":string, "standard output"=w4821:string)  [unwired: 4 in, 2 out]
                "standard output 2" <- w4821
                n3879 = Match Pattern(string=w4821, regular expression="JSONH Check String") -> (match substring=w4819:string, offset past match=w4818:i32)  [unwired: 1 in, 2 out]
                n3880 = Equal?(x=w4819, y="JSONH Check String") -> (x = y?=→"Upload \nConfirmed 2":bool)
              }
            }
            n3881 = Divide(x=w4661, y=3600.0 ("f")) -> (x/y=w4654:dbl)
            n3882 = local read "run time"() -> (w4711:string[])
            n3883 = Round To Nearest(number=w4654) -> (nearest integer value=w4653:dbl)
            n3884 = Number To Decimal String(number=w4653) -> (decimal integer string=w4652:string)  [unwired: 1 in]
            n3885 = Index Array(array="Sensor Information", index (col) #1=0 ("disabled index (col)"), index (col) #2=1 ("index (col)"), index (col) #3=2 ("index (col)"), index (col) #4=3 ("index (col)")) -> (element #1=→"Sensor name":string[], element #2=→"model num":string[], element #3=→"run time":string[], element #4=→"state":string[])  [unwired: 4 in]
            n3886 = Insert Into Array(array=w4711, index=1, new element #1=w4652, new element #2=w4652, new element #3=w4652, new element #4=w4652, new element #5=w4652, new element #6=w4652) -> (w4676:string[])
            "run" <- w4676
            n3887 = local read "out"() -> (w4658:string[])
            n3888 = local read "Sensor Information"() -> (w4678:string[][])
            n3889 = Replace Array Subset(array=w4678, new element #1=w4676, index (col) #1=2 ("disabled index (col)"), new element #2=w4658, index (col) #2=3 ("index (col)")) -> (w4677:string[][])  [unwired: 2 in]
            n3890 = local write "Sensor Information"(w4677) -> ()
          }
        }
        n3891 = case shown="True" w4625 {
          frame False {
          }
          frame True {
            n3892 = Equal?(x="FLAG", y=0.0) -> (x = y?=w4642:bool)
            n3893 = case shown="False" w4642 {
              frame False {
                n3894 = Get Date/Time In Seconds() -> (seconds since 1Jan1904=w4648:timestamp)
                n3895 = local read "START 2"() -> (w4646:dbl)
                n3896 = To Double Precision Float(number=w4648) -> (double precision float=w4647:dbl)
                n3897 = Subtract(x=w4647, y=w4646) -> (x-y=→"SENSOR TIME  2":dbl)
              }
              frame True {
                n3898 = Get Date/Time In Seconds() -> (seconds since 1Jan1904=w4650:timestamp)
                n3899 = To Double Precision Float(number=w4650) -> (double precision float=→"START 2":dbl)
                n3900 = local write "FLAG"(100.0 ("FLAG")) -> ()
              }
            }
          }
        }
        n3901 = disable-structure shown="Disabled" {
          disable-tunnel: w4628 -> [w4637 _]
          disable-tunnel: [w4636 _] -> w4627
          frame Disabled {
            n3902 = local read "Json St Flg"() -> (w4635:bool)
            n3903 = case shown="True" w4635 {
              tunnel: w4637 -> [w4638 w4640]
              tunnel: [w4638 w4639] -> w4636
              frame False {
              }
              frame True {
                n3904 = Increment(x=w4640) -> (x+1=w4639:dbl)
                "T cycle" <- w4639
                n3905 = local write "Json St Flg"(FALSE ("Json St Flg")) -> ()
              }
            }
          }
          frame Enabled {
          }
        }
        n3906 = local read "Quit"() -> (w4622:bool)
      }
    }
    frame Enabled {
    }
  }
  n3907 = stacked-sequence {
    tunnel: [w5020] -> w38
    frame #0 {
      w5020 = FALSE ("Upload \nConfirmed")
      n3908 = local write "Upload \nConfirmed"(w5020) -> ()
      n3909 = local write "St Str"("") -> ()
    }
  }
  n3910 = disable-structure shown="Disabled" {
    disable-tunnel: w38 -> [w5021 _]
    frame Disabled {
      n3911 = case shown="True" {
        selector: _ -> [_ _]
        tunnel: w5021 -> [_ w5022]
        frame False {
        }
        frame True {
          n3912 = while {
            tunnel: [w5028] -> _
            tunnel: w5022 -> [_]
            i -> [w5028]
            stop <- w5023 stop-if-true
            n3913 = local read "Json End Flg"() -> (w5027:bool)
            n3914 = Wait (ms)(milliseconds to wait=u32 20 ("Refresh Rate (ms)")) -> ()  [unwired: 1 out]
            n3915 = local read "refresh flag"() -> (w5024:bool)
            n3916 = local read "RUN"() -> (w5025:bool)
            n3917 = And(x=w5025, y=w5024) -> (x .and. y?=w5026:bool)
            n3918 = Or(x=w5026, y=w5027) -> (x .or. y?=w5029:bool)
            "AR Led" <- w5029
            n3919 = case shown="True" w5029 {
              frame False {
              }
              frame True {
                w5046 = "\",\""
                n3920 = local read "UUID"() -> (w5044:string)
                n3921 = local write "refresh flag"(FALSE ("refresh flag")) -> ()
                n3922 = local read "time"() -> (w5033:dbl)
                n3923 = Multiply(x=w5033, y=60.0) -> (x*y=w5032:dbl)
                n3924 = Concatenate Strings("UUID\" : \"", w5044, "\"}") -> (w5047:string)
                n3925 = Number To Fractional String(number=w5032, width (-)=i16 10, precision (6)=i16 4) -> (F-format string=w5061:string)  [unwired: 1 in]
                n3926 = Concatenate Strings("{", "\"Time\":\"", w5061, w5046) -> (w5056:string)
                n3927 = stacked-sequence {
                  tunnel: w5046 -> [w5109 w5117 w5124 w5132 w5140 w5149 w5156]
                  tunnel: [w5110 _ _ _ _ _ _] -> w5060
                  tunnel: [_ w5118 _ _ _ _ _] -> w5059
                  tunnel: [_ _ w5125 _ _ _ _] -> w5058
                  tunnel: [_ _ _ w5134 _ _ _] -> w5057
                  tunnel: w5047 -> [_ _ _ _ _ _ w5167]
                  tunnel: [_ _ _ _ _ _ w5166] -> w5043
                  tunnel: [_ _ _ _ _ w5146 _] -> w5042
                  tunnel: [_ _ _ _ w5139 _ _] -> w5041
                  frame #0 {
                    n3928 = local read "NORMAL LOAD"() -> (w5108:dbl)
                    n3929 = Number To Fractional String(number=w5108, width (-)=i16 10, precision (6)=i16 4) -> (F-format string=w5111:string)  [unwired: 1 in]
                    n3930 = Concatenate Strings("NormalLoad\":\"", w5111, w5109) -> (w5110:string)
                  }
                  frame #1 {
                    n3931 = local read "Temp"() -> (w5116:dbl)
                    n3932 = Number To Fractional String(number=w5116, width (-)=i16 10, precision (6)=i16 4) -> (F-format string=w5119:string)  [unwired: 1 in]
                    n3933 = Concatenate Strings("Temperature\":\"", w5119, w5117) -> (w5118:string)
                  }
                  frame #2 {
                    n3934 = local read "cof"() -> (w5122:dbl)
                    n3935 = Number To Fractional String(number=w5122, width (-)=i16 10, precision (6)=i16 4) -> (F-format string=w5126:string)  [unwired: 1 in]
                    n3936 = Concatenate Strings("FrictionalForce\":\"", w5126, w5124) -> (w5125:string)
                  }
                  frame #3 {
                    n3937 = local read "Set Hz"() -> (w5130:dbl)
                    n3938 = Multiply(x=w5130, y=60.0) -> (x*y=w5129:dbl)
                    n3939 = Number To Fractional String(number=w5129, width (-)=i16 10, precision (6)=i16 4) -> (F-format string=w5135:string)  [unwired: 1 in]
                    n3940 = Concatenate Strings("Speed\":\"", w5135, w5132) -> (w5134:string)
                  }
                  frame #4 {
                    n3941 = local read item#-1() -> (w5138)
                    n3942 = Number To Fractional String(number=w5138, width (-)=i16 10, precision (6)=i16 4) -> (F-format string=w5142:string)  [unwired: 1 in]
                    n3943 = Concatenate Strings("LinearDeformation\":\"", w5142, w5140) -> (w5139:string)
                  }
                  frame #5 {
                    n3944 = local read "AIR TEMP"() -> (w5145:dbl)
                    n3945 = local read "Json St Flg"() -> (w5147:bool)
                    n3946 = local read "Json End Flg"() -> (w5148:bool)
                    n3947 = Number To Fractional String(number=w5145, width (-)=i16 10, precision (6)=i16 4) -> (F-format string=w5151:string)  [unwired: 1 in]
                    n3948 = Concatenate Strings("Vibration\":\"", w5151, w5149) -> (w5146:string)
                    n3949 = And(x=w5147, y=w5148) -> ()  [unwired: 1 out]
                  }
                  frame #6 {
                    n3950 = local read "Json End Flg"() -> (w5155:bool)
                    n3951 = Get Date/Time In Seconds() -> (seconds since 1Jan1904=w5163:timestamp)
                    n3952 = local read "Json St Flg"() -> (w5154:bool)
                    n3953 = To Double Precision Float(number=w5163) -> (double precision float=w5162:dbl)
                    n3954 = Subtract(x=w5162, y=2082844800.0) -> (x-y=w5160:dbl)
                    n3955 = Number To Fractional String(number=w5160, width (-)=i16 12, precision (6)=i16 0) -> (F-format string=w5157:string)  [unwired: 1 in]
                    n3956 = case shown="True" w5155 {
                      tunnel: ["" w5170] -> w5164
                      tunnel: w5157 -> [_ w5171]
                      tunnel: w5156 -> [_ w5169]
                      frame False {
                      }
                      frame True {
                        n3957 = local write "Json End Flg"(FALSE ("Json St Flg")) -> ()
                        n3958 = Concatenate Strings("End\": \"", w5171, w5169) -> (w5170:string)
                      }
                    }
                    n3959 = case shown="True" w5154 {
                      tunnel: [w5174 w5177] -> w5165
                      tunnel: w5157 -> [_ w5178]
                      tunnel: w5156 -> [_ w5175]
                      frame False {
                        n3960 = local read "St Str"() -> (w5174:string)
                      }
                      frame True {
                        n3961 = Concatenate Strings("Start\":\"", w5178, w5175) -> (w5177:string)
                        "St Str" <- w5177
                        n3962 = local write "Json St Flg"(FALSE ("Json St Flg")) -> ()
                      }
                    }
                    n3963 = Concatenate Strings(w5165, w5164, w5167) -> (w5166:string)
                  }
                }
                n3964 = local read "FILE"() -> (w5035:string)
                n3965 = Concatenate Strings("\",\"OperatorID\":\"" ("string"), "Operator ID") -> (w5038:string)
                n3966 = Concatenate Strings("\",\"DatasetTitle\":\"" ("string"), w5035) -> (w5037:string)
                n3967 = Concatenate Strings("\",\"SerialNumber\":\"" ("string"), "Serial No") -> (w5067:string)
                n3968 = Concatenate Strings("\",\"ModelNumber\":\"" ("string"), "Model No") -> (w5066:string)
                n3969 = Concatenate Strings(w5067, w5066) -> (w5049:string)
                n3970 = Concatenate Strings("{\"SecretKey\":\"", "Secret Key", w5049, w5038, w5037, "\",\"Samples\":[") -> (w5054:string)
                n3971 = Concatenate Strings(w5056, w5060, w5059, w5058, w5057, w5041, w5042, w5043) -> (w5055:string)
                n3972 = Concatenate Strings(w5054, w5055, "]}") -> (w5053:string)
                n3973 = stacked-sequence {
                  tunnel: w5053 -> [w5082 _ _]
                  tunnel: [_ _ w5099] -> _
                  frame #0 {
                    (unwired) FALSE ("convert eol (F)")
                    w5084 = enum16{"start", "end", "current"}."start" ("pos mode (0:2)")
                    n3974 = Path To String(path="Path") -> (string=w5090:string)
                    n3975 = Concatenate Strings(w5090, "\\", "Data File Name") -> (w5092:string)
                    n3976 = local write "standard output"(" ") -> ()
                    n3977 = String To Path(string=w5092) -> (path=w5081:path)
                    n3978 = call <vilib>:"Open_Create_Replace File.vi"("advisory dialog? (display:T)"=FALSE, "function (open:0)"=T32."create or replace", "file path"=w5081) -> ("error out"=w5095:errorcluster, "refnum"=w5094:refnum<file>)  [unwired: 5 in, 2 out]
                    n3979 = Set File Position(refnum=w5094, from (0:start)=w5084, error in=w5095) -> (refnum out=w5075:refnum<file>, error out=w5074:errorcluster)  [unwired: 1 in]
                    n3980 = Write to Binary File(file (use dialog)=w5075, data=" ", error in=w5074, 5:FALSE ("prepend array or string size? (T)")) -> (refnum out=w5085:refnum<file>, error out=w5086:errorcluster)  [unwired: 2 in, 1 out]
                    n3981 = Set File Position(offset (in bytes) (0)=w5084, refnum=w5085, error in=w5086) -> (refnum out=w5078:refnum<file>, error out=w5077:errorcluster)  [unwired: 1 in]
                    n3982 = Write to Binary File(file (use dialog)=w5078, data=w5082, error in=w5077, 5:FALSE ("prepend array or string size? (T)")) -> (error out=w5080:errorcluster)  [unwired: 2 in, 2 out]
                    n3983 = flat-sequence {
                      tunnel: w5081 -> [w5097]
                      tunnel: w5080 -> [_]
                      frame #0 {
                        n3984 = call <vilib>:"Read Characters From File.vi"("file path (dialog if empty)"=w5097) -> ("character string"=→"JSON string":string)  [unwired: 5 in, 3 out]
                      }
                    }
                    "SinglePoint" <- w5082
                  }
                  frame #1 {
                  }
                  frame #2 {
                    (unwired) "\"Stored\": true" ("string")
                    n3985 = call <vilib>:"System Exec.vi"("run minimized? (F)"=TRUE, "wait until completion? (T)"=TRUE, "working directory"=path "C:/LAB-IQ-NXT", "command line"="C:\\LAB-IQ-NXT\\JPost.bat") -> ("standard error"=→"Respose From Server":string, "standard output"=w5102:string)  [unwired: 4 in, 2 out]
                    "standard output" <- w5102
                    n3986 = Match Pattern(string=w5102, regular expression="JSON Check String") -> (match substring=w5100:string, offset past match=w5099:i32)  [unwired: 1 in, 2 out]
                    n3987 = Equal?(x=w5100, y="JSON Check String") -> (x = y?=→"Upload \nConfirmed":bool)
                  }
                }
              }
            }
            n3988 = local read "Quit"() -> (w5023:bool)
          }
        }
      }
    }
    frame Enabled {
    }
  }
  n3989 = disable-structure shown="Disabled" {
    disable-tunnel: _ -> [w5185 _]
    frame Disabled {
      n3990 = while {
        shift-right: [w5193] -> w5181
        shift-left: _ -> [w5194]
        shift-right: [w5191] -> w5182
        shift-left: errorcluster {"status"=TRUE, "code"=0, "source"="Init"} ("error out") -> [w5192]
        shift-right: [w5189] -> _
        shift-left: "" -> [w5190]
        tunnel: [w5187] -> _
        tunnel: w5185 -> [_]
        i -> [w5187]
        stop <- w5186 stop-if-true
        n3991 = flat-sequence {
          tunnel: [w5195] -> w5188
          frame #0 {
            n3992 = Wait (ms)(milliseconds to wait=10.0 ("Delay")) -> (millisecond timer value=w5195:u32)
          }
        }
        n3993 = case shown="No Error" w5192 {
          selector: w5192 -> [w5225 w5344]
          tunnel: [w5208 w5346] -> w5193
          tunnel: [w5207 w5345] -> w5191
          tunnel: w5194 -> [w5226 w5338]
          tunnel: w5190 -> [w5206 w5337]
          tunnel: [w5205 w5337] -> w5189
          tunnel: w5188 -> [_ _]
          frame No Error {
            n3994 = Concatenate Strings("\r", "\n") -> (w5217:string)  [unwired: 1 in]
            n3995 = case shown="True" w5218 {
              tunnel: w5226 -> [w5250 w5257]
              tunnel: w5225 -> [w5249 w5256]
              tunnel: [w5250 w5255] -> w5224
              tunnel: [w5249 w5254] -> w5204
              tunnel: w5217 -> [_ w5253]
              frame False {
              }
              frame True {
                n3996 = VISA Write(VISA resource name=w5257, write buffer=w5253, error in (no error)=w5256) -> (VISA resource name out=w5255:refnum<visa-resource-name>, error out=w5254:errorcluster)  [unwired: 1 out]
                n3997 = local write "Read String"("") -> ()
                n3998 = local write item#-1(FALSE) -> ()
              }
            }
            n3999 = property class="Instr"(reference=w5224, error in=w5204) -> (reference out=w5223:refnum<visa-resource-name>, error out=w5222:errorcluster, "Serial Settings:Number of Bytes at Serial Port"=w5221:u32)
            n4000 = Greater?(x=w5221, y=u32 100) -> (0:w5219:bool)
            n4001 = case shown="True" w5219 {
              tunnel: w5223 -> [w5260 w5284]
              tunnel: w5222 -> [w5259 w5283]
              tunnel: w5221 -> [_ w5282]
              tunnel: [w5260 w5281] -> w5210
              tunnel: [w5259 w5280] -> w5209
              tunnel: w5206 -> [w5258 w5279]
              tunnel: [w5258 ""] -> w5205
              frame False {
              }
              frame True {
                w5269 = u32 6 ("y")
                # "Page 84 of \nmanual"
                n4002 = VISA Read(VISA resource name=w5284, byte count=w5282, error in (no error)=w5283) -> (VISA resource name out=w5281:refnum<visa-resource-name>, read buffer=w5277:string, error out=w5280:errorcluster)  [unwired: 1 out]
                n4003 = while {
                  tunnel: w5277 -> [w5333]
                  tunnel: [w5329] -> w5271 mode=indexing
                  tunnel: [w5323] -> w5275 mode=indexing
                  tunnel: [w5321] -> _
                  i -> [w5321]
                  stop <- w5326 stop-if-true
                  n4004 = String Subset(string=w5333, offset (0)=w5321) -> (substring=w5328:string)  [unwired: 1 in]
                  n4005 = String To Byte Array(string=w5328) -> (unsigned byte array=w5332:u8[])
                  n4006 = String Length(string=w5328) -> (length=w5327:i32)
                  n4007 = Index Array(array=w5332) -> (element=w5331:u8)  [unwired: 1 in]
                  n4008 = Equal To 0?(x=w5327) -> (x = 0?=w5326:bool)
                  n4009 = Number To Boolean Array(number=w5331) -> (Boolean array=w5325:bool[])
                  n4010 = Reverse 1D Array(array=w5325) -> (reversed array=w5324:bool[])
                  n4011 = And(x=w5325, y=bool[] [FALSE, FALSE, FALSE, FALSE, FALSE, FALSE, TRUE, TRUE] ("Boolean array")) -> (x .and. y?=w5329:bool[])
                  n4012 = And(x=w5324, y=bool[] [FALSE, FALSE, TRUE, TRUE, TRUE, TRUE, TRUE, TRUE] ("Boolean array")) -> (x .and. y?=w5323:bool[])
                }
                n4013 = Concatenate Strings(w5279, w5277) -> (→"Read String":string)
                n4014 = while {
                  tunnel: w5271 -> [w5320] mode=indexing
                  tunnel: [w5316] -> w5274
                  i -> [w5316]
                  stop <- w5317 stop-if-true
                  n4015 = Search 1D Array(1D array=w5320, element=TRUE) -> (index of element=w5318:i32)  [unwired: 1 in]
                  n4016 = Less Than 0?(x=w5318) -> (x < 0?=w5317:bool)
                }
                n4017 = Delete From Array(array=w5275, length=w5274, index (row)=0) -> (array with subset deleted=w5270:bool[][])  [unwired: 1 in, 1 out]
                n4018 = Array Size(array=w5270) -> (size(s)=w5272:i32[])
                n4019 = Index Array(array=w5272) -> (element=w5264:i32)  [unwired: 1 in]
                n4020 = Greater?(x=w5264, y=w5269) -> (0:w5267:bool)
